vi "FB_initialize.vi"() -> (0 "error out":errorcluster, 1 "Transformed Calibration Matrix":dbl[][](array[numeric]), 3 "FB out":refnum<k21>)   [LabVIEW 2021]
uses:
  <vilib>/DAQmx/create/channels.llb/DAQmx Create Channel (AI-Voltage-Basic).vi
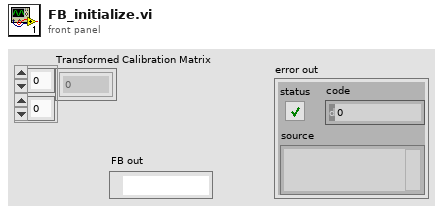
[diagram p1: front panel]
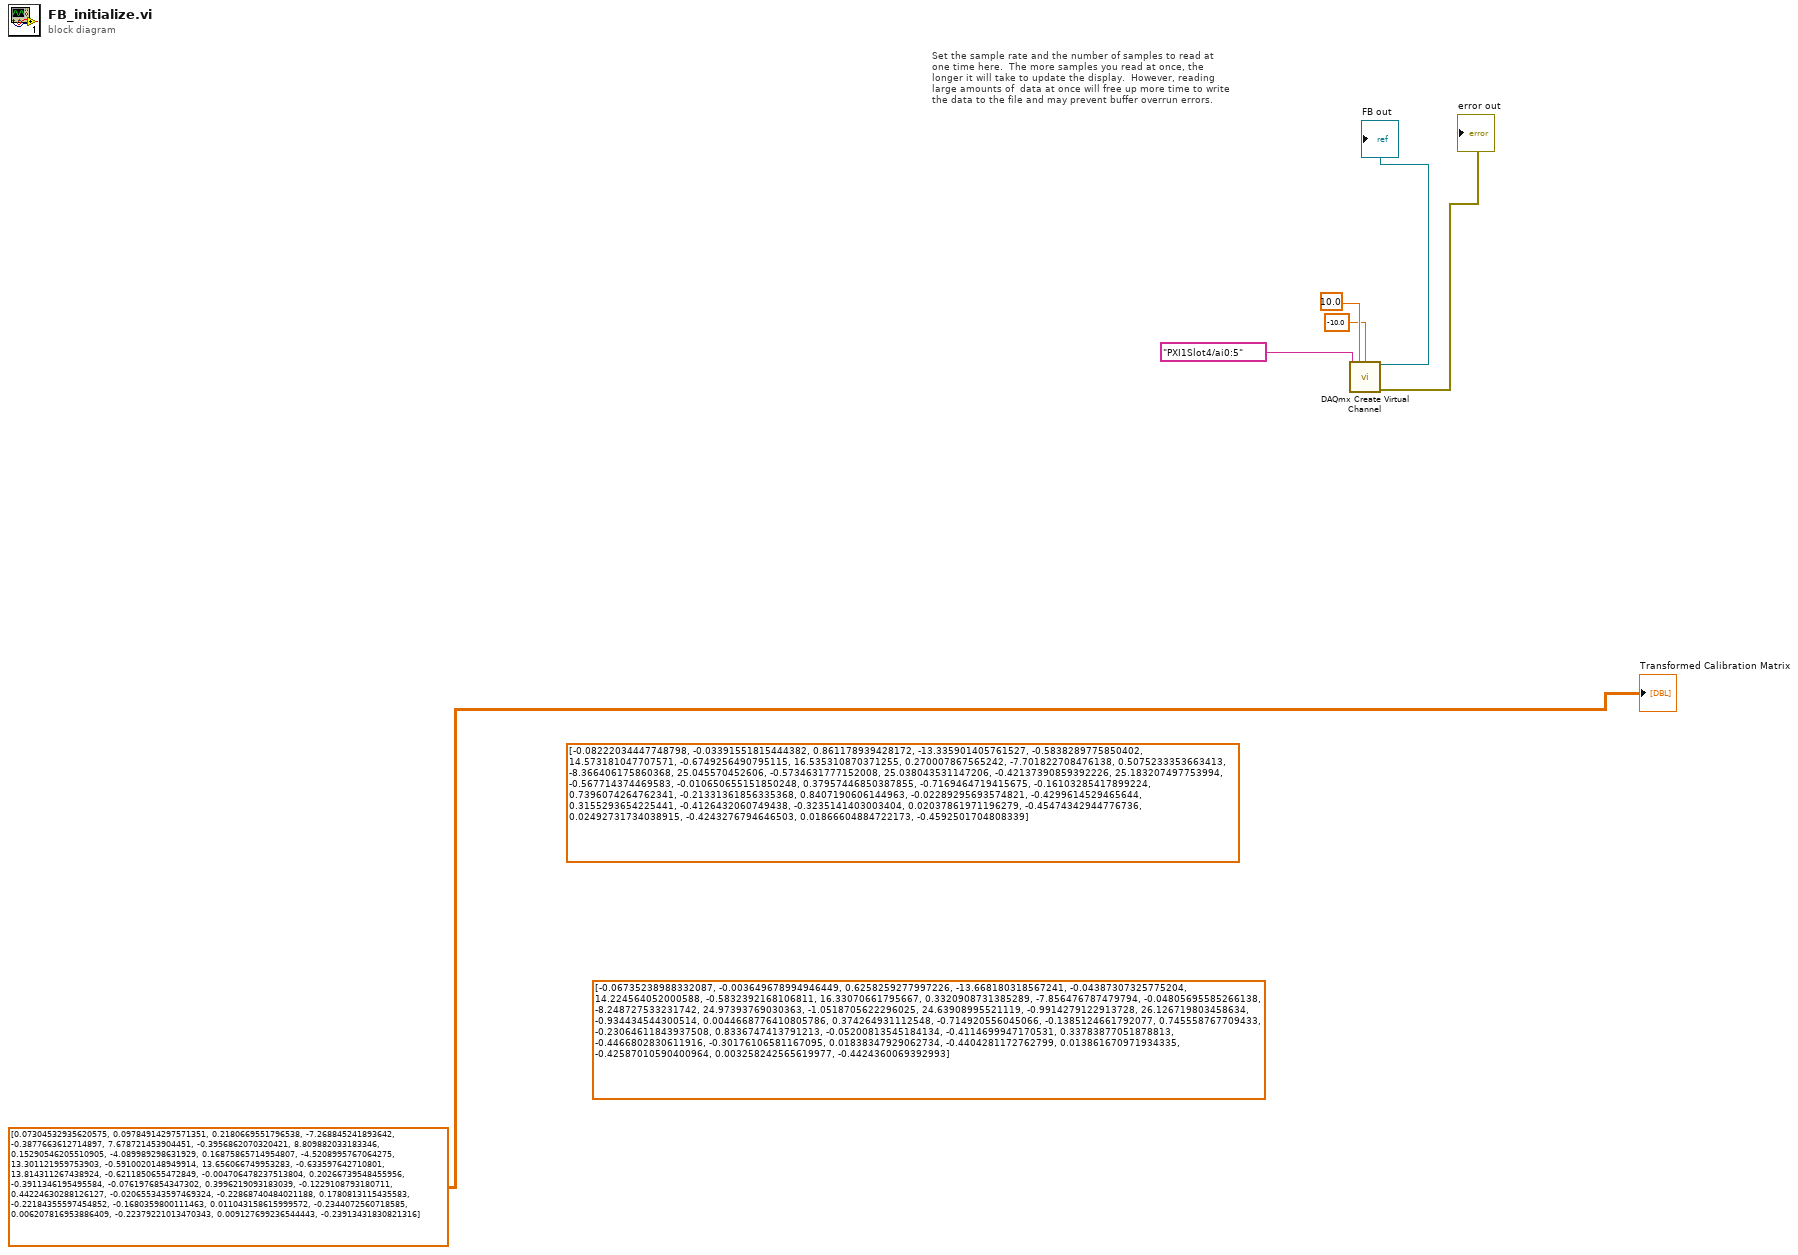
[diagram p0: block diagram]
diagram:
  (unwired) dbl[][] [[-0.08222034447748798, -0.03391551815444382, 0.861178939428172, -13.335901405761527, -0.5838289775850402, 14.573181047707571], [-0.6749256490795115, 16.535310870371255, 0.270007867565242, -7.701822708476138, 0.5075233353663413, -8.366406175860368], [25.045570452606, -0.5734631777152008, 25.038043531147206, -0.42137390859392226, 25.183207497753994, -0.567714374469583], [-0.010650655151850248, 0.37957446850387855, -0.7169464719415675, -0.16103285417899224, 0.7396074264762341, -0.21331361856335368], [0.8407190606144963, -0.02289295693574821, -0.4299614529465644, 0.3155293654225441, -0.4126432060749438, -0.3235141403003404], [0.02037861971196279, -0.45474342944776736, 0.02492731734038915, -0.4243276794646503, 0.01866604884722173, -0.4592501704808339]] ("Calibration Matrix")
  (unwired) dbl[][] [[-0.06735238988332087, -0.003649678994946449, 0.6258259277997226, -13.668180318567241, -0.04387307325775204, 14.224564052000588], [-0.5832392168106811, 16.33070661795667, 0.3320908731385289, -7.856476787479794, -0.04805695585266138, -8.248727533231742], [24.97393769030363, -1.0518705622296025, 24.63908995521119, -0.9914279122913728, 26.126719803458634, -0.934434544300514], [0.0044668776410805786, 0.374264931112548, -0.714920556045066, -0.1385124661792077, 0.745558767709433, -0.23064611843937508], [0.8336747413791213, -0.05200813545184134, -0.4114699947170531, 0.33783877051878813, -0.4466802830611916, -0.30176106581167095], [0.01838347929062734, -0.4404281172762799, 0.013861670971934335, -0.42587010590400964, 0.003258242565619977, -0.4424360069392993]] ("Calibration Matrix")
  # "Set the sample rate and the number of samples to read at\none time here.  The more samples you read at once, the\nlonger it will take to update the display.  However, reading\nlarge amounts of  data at once will free up more time to write\nthe data to the file and may prevent buffer overrun errors."
  n1 = call-poly <vilib>:"DAQmx Create Virtual Channel.vi"("maximum value"=10.0, "minimum value"=-10.0, "physical channels"=tag "PXI1Slot4/ai0:5") -> ("task out"=→"FB out":refnum<k21>, "error out"=→"error out":errorcluster)  [unwired: 11 in]
  "Transformed Calibration Matrix" <- dbl[][] [[0.07304532935620575, 0.09784914297571351, 0.2180669551796538, -7.268845241893642, -0.3877663612714897, 7.678721453904451], [-0.3956862070320421, 8.809882033183346, 0.15290546205510905, -4.089989298631929, 0.16875865714954807, -4.5208995767064275], [13.301121959753903, -0.5910020148949914, 13.656066749953283, -0.633597642710801, 13.814311267438924, -0.6211850655472849], [-0.004706478237513804, 0.20266739548455956, -0.3911346195495584, -0.0761976854347302, 0.3996219093183039, -0.1229108793180711], [0.44224630288126127, -0.020655343597469324, -0.22868740484021188, 0.1780813115435583, -0.22184355597454852, -0.1680359800111463], [0.011043158615999572, -0.2344072560718585, 0.006207816953886409, -0.22379221013470343, 0.009127699236544443, -0.23913431830821316]] ("Calibration Matrix")
